vi "Initialize.vi"(7 "Micropulse # In":i32, 8 "error in (no error)":errorcluster, 9 "Hard Reset?":bool caption="Hard Reset? (def: F - Soft Reset)", 10 "Sample Frequency":T1, 11 "TCP config":T2={"Connection ID"=refnum, "IP address"="10.1.1.2", "host port"=1067, "OC timeout"=-1, "Read timeout"=0, "Write timeout"=0} {"Write timeout" format="%dms"; "Read timeout" format="%dms"; "OC timeout" format="%dms"}) -> (0 "error out":errorcluster, 5 "Micropulse # Out":i32)   [LabVIEW 2026, in "MicroPulse_Driver.lvlib"]
doc: "Establishes communication with the instrument and optionally performs an instrument identification query and/or an instrument reset. It also places the instrument in a default state needed for other instrument driver operations. Therefore, call this VI before calling other instrument driver VIs for this instrument. Generally, you need to call the <b>Initialize</b> VI only once at the beginning of an application."
uses:
  MicroPulse_Driver.lvlib
  Data/Datatypes/TCP config.ctl
  Data/Datatypes/MP - sample frequency.ctl
  Private/MP-Registry Action-Enum.ctl
  <instrlib>/MicroPulse/Public/Data/Datatypes/MP - encoder mode.ctl
panel:
  # "(c) 2014 <Enter Company Name Here>.  ALL RIGHTS RESERVED."
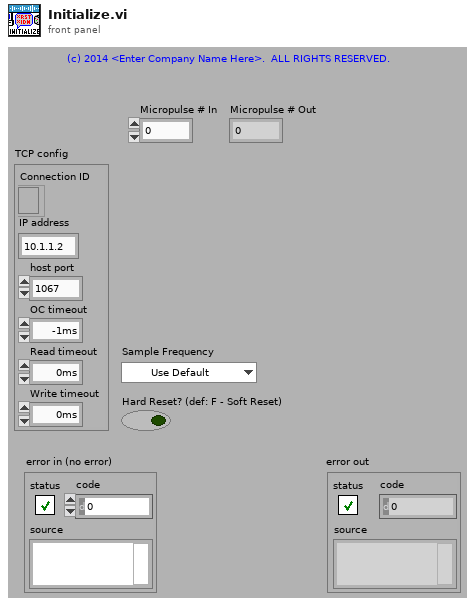
[diagram p1: front panel]
types:
  T1 = typedef "MicroPulse_Driver.lvlib/MP - sample frequency.ctl" = enum16{"Use Default", "200MHz (LT2 only)", "100MHz", "50MHz", "25MHz", "10MHz"}
  T2 = typedef "MicroPulse_Driver.lvlib/TCP config.ctl" = cluster{"Connection ID":refnum<k5>, "IP address":string, "host port":u16, "OC timeout":i32, "Read timeout":i32, "Write timeout":i32}
  T3 = typedef "MicroPulse_Driver.lvlib/MP-Registry Action-Enum.ctl" = enum16{"Read", "Add Test", "Add Command", "Add Gate Command", "Add Encoder Command", "Clear Command  List", "Set Registry", "Set System Details", "Set DOF", "Set Velocity", "Disable Asynch Reads", "Enable Asynch Reads", "Add Connection", "Disconnect", "Shutdown"}
  T4 = typedef "MicroPulse_Driver.lvlib/MP - general system status.ctl" = cluster{"System Type":T5, "Serial No.":u64, "Channels":cluster{"Conv":u8, "PA":u16, "Extra":u32}, "Sample Frequency":cluster{"Default":u8, "Actual":u8}, "Software Versions":string, "Data Output Format":cluster{"Default":T6, "Actual":T6}, "Temperatures":cluster{"System":u8, "Processor":u8, "Slave Sys":u8, "Slave Proc":u8}, "Tx Buffer Size":u32, "System Error":string, "No. of Cards":u8, "DAC Gain":i16, "Uptimes":cluster{"since Power":u32, "since RSTS":u32, "since SRST":u32}, "Voltages":cluster{"Nominal":dbl, "Measured":dbl, "Difference":dbl}[], "Interface Cards":T7[]}
  T5 = typedef "MicroPulse_Driver.lvlib/MP - instrument type.ctl" = enum16{"MicroPulse 5", "LT1", "LT2", "LTPA", "MPLT", "MicroPulse 6", "PipeScanner", "<MicroPulse>", "Micropulse 4", "Simulated Data"}
  T6 = typedef "MicroPulse_Driver.lvlib/MP - data output format.ctl" = enum16{"", "8-bit Mode", "10-bit Mode", "12-bit Mode", "16-bit Mode", "8-bit Log Mode", "12-bit Packed Mode"}
  T7 = typedef "MicroPulse_Driver.lvlib/MP - interface card status.ctl" = cluster{"Status":u8, "Map":u8, "Board - T":u8, "FPGA - T":u8, "PAIF Status":string, "Version":string}
  T8 = typedef "MicroPulse_Driver.lvlib/MP - encoder mode.ctl" = enum16{"24-bit + LCI", "32-bit + LCI", "32-bit + LLC", "24-bit + STS6", "32-bit + STS6", "32-bit + LLC+STS6"}
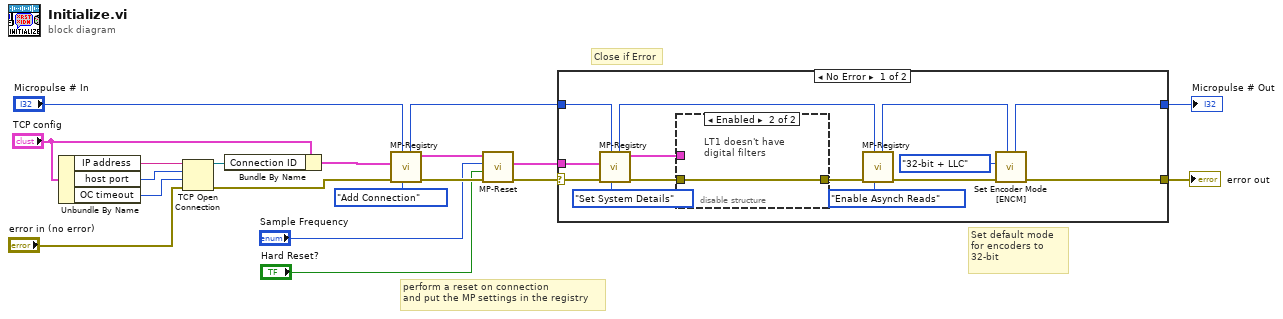
[diagram p0: block diagram]
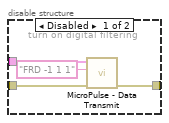
[diagram p2: hidden frame]
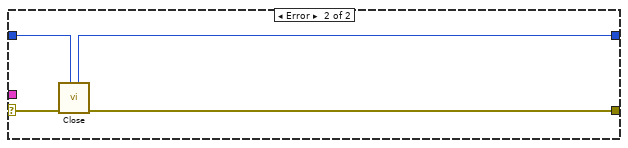
[diagram p3: hidden frame]
diagram:
  # "perform a reset on connection\nand put the MP settings in the registry"
  # "Set default mode for encoders to 32-bit"
  # "Close if Error"
  n1 = Unbundle By Name("TCP config") -> ("IP address"=w11:string, "host port"=w12:u16, "OC timeout"=w13:i32)
  n2 = TCP Open Connection(address=w11, remote port or service name=w12, timeout ms (60000)=w13, error in (no error)="error in (no error)") -> (connection ID=w14:refnum<k5>, error out=w4:errorcluster)  [unwired: 1 in]
  n3 = Bundle By Name(cluster="TCP config", "Connection ID"=w14) -> (w8:T2)
  n4 = call "MP-Registry.vi"("Action"=MP-Registry_Action-Enum."Add Connection", "Micropulse # In"="Micropulse # In", "error in (no error)"=w4, "Data in"=w8) -> ("error out"=w7:errorcluster, "TCP config"=w5:T2, "Micropulse # Out"=w15:i32)  [unwired: 4 in, 1 out]
  n5 = call "MP-Reset.vi"("error in (no error)"=w7, "Hard Reset?"="Hard Reset?", "Sample Frequency"="Sample Frequency", "TCP config"=w5) -> ("error out"=w6:errorcluster, "System Status"=w3:T4)  [unwired: 5 in, 1 out]
  n6 = case shown="No Error" w6 {
    selector: w6 -> [w33 w41]
    tunnel: [w23 w42] -> w19
    tunnel: [w20 w40] -> w16
    tunnel: w15 -> [w30 w39]
    tunnel: w3 -> [w31 _]
    frame No Error {
      n7 = call "MP-Registry.vi"("Action"=MP-Registry_Action-Enum."Set System Details", "Micropulse # In"=w30, "error in (no error)"=w33, "Data in"=w31) -> ("error out"=w29:errorcluster, "TCP config"=w28:T2, "Micropulse # Out"=w25:i32)  [unwired: 4 in, 1 out]
      n8 = disable-structure shown="Enabled" {
        disable-tunnel: w29 -> [w37 w38]
        disable-tunnel: [w36 w38] -> w27
        disable-tunnel: w28 -> [w34 _]
        frame Disabled {
          # "turn on digital filtering"
          n9 = call "MicroPulse - Data Transmit.vi"("error in (no error)"=w37, "data"="FRD -1 1 1", "TCP config"=w34) -> ("error out"=w36:errorcluster)  [unwired: 6 in, 2 out]
        }
        frame Enabled {
          # "LT1 doesn't have digital filters"
        }
      }
      n10 = call "MP-Registry.vi"("Action"=MP-Registry_Action-Enum."Enable Asynch Reads", "Micropulse # In"=w25, "error in (no error)"=w27) -> ("error out"=w24:errorcluster, "Micropulse # Out"=w21:i32)  [unwired: 5 in, 2 out]
      n11 = call <instrlib>:"Set Encoder Mode [ENCM].vi"("Micropulse # In"=w21, "error in (no error)"=w24, "Encoder Mode"=MP_-_encoder_mode."32-bit + LLC") -> ("error out"=w23:errorcluster, "Micropulse # Out"=w20:i32)  [unwired: 7 in]
    }
    frame Error {
      n12 = call "Close.vi"("Micropulse # In"=w39, "error in (no error)"=w41) -> ("error out"=w42:errorcluster, "Micropulse # Out"=w40:i32)  [unwired: 8 in]
    }
  }
  "error out" <- w19
  "Micropulse # Out" <- w16
